vi "3.2.1-VectorNav WaitForReply.vi"(10 "error in":errorcluster, 11 "FPGA Ref In":T1) -> (2 "error out":errorcluster, 3 "FPGA Ref Out":T1)   [LabVIEW 2010]
doc: "In order for on-demand sampling to work, it's important that the cRIO and FPGA both agree on whether the FPGA should currently be sampling. This VI uses boolean flags to ensure that the FPGA knows when it's supposed to be sampling and that the cRIO knows when the FPGA is done so it can go grab the reply out of the Read FIFO."
uses:
  2-Low Neurons/2-FPGA VI Typedef.ctl
  2-Low Neurons/2.7-Sense Queries Typedef.ctl
  <vilib>/rvi/interface/nirviReadWriteControl/nirviReadWriteControl.xnode
  FPGA Bitfiles/DaveBrain_FPGATarget_1-Hindbrain_F0E489D8.lvbitx
  1-Hindbrain.vi
  <vilib>/rvi/interface/common/niFpgaNodeNameForErrorReporting.ctl
  <vilib>/rvi/errors/niLvFpgaWhatHappensToTopLevelVI.ctl
  2-Low Neurons/2.4-How Sensor Typedef.ctl
  <vilib>/Utility/error.llb/Error Cluster From Error Code.vi
  <vilib>/rvi/errors/niLvFpgaAdjustHostInterfaceError.vi
  3.0-Global.vi
  NiFpgaLv.dll
panel:
  out "VectorNav Ack Query":bool=TRUE
  out "VectorNav Cmd Query":bool=TRUE
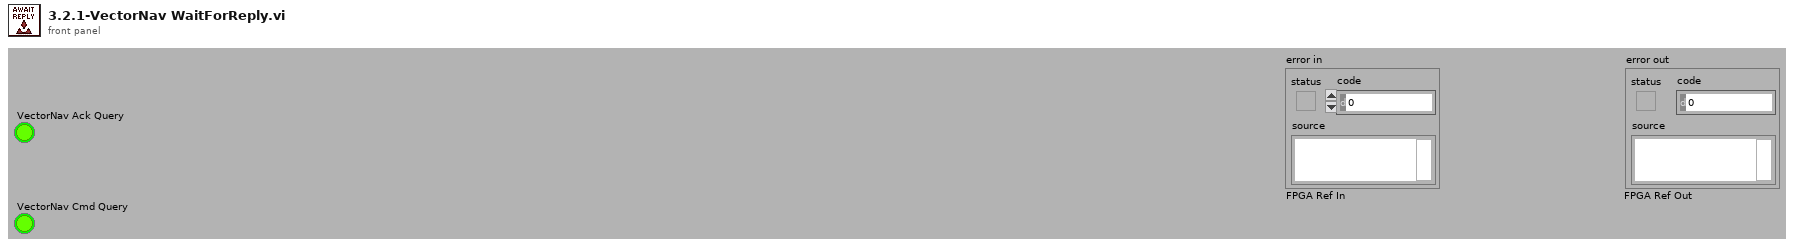
[diagram p1: front panel]
types:
  T1 = typedef "2-FPGA VI Typedef.ctl" = refnum<k20>
  T2 = typedef "2.7-Sense Queries Typedef.ctl" = cluster{"VectorNav Query":bool}
  T3 = typedef "niFpgaNodeNameForErrorReporting.ctl" = enum16{"Open FPGA VI Reference", "Read/Write Control", "Invoke Method: Abort", "Invoke Method: Acknowledge IRQ", "Invoke Method: Download", "Invoke Method: FIFO.Configure", "Invoke Method: FIFO.Read", "Invoke Method: FIFO.Start", "Invoke Method: FIFO.Stop", "Invoke Method: FIFO.Write", "Invoke Method: Reset", "Invoke Method: Run", "Invoke Method: Wait on IRQ", "Close FPGA VI Reference"}
  T4 = typedef "niLvFpgaWhatHappensToTopLevelVI.ctl" = enum16{"top level VI scripted behind XNode", "top level VI inlined behind XNode"}
  T5 = typedef "2.4-How Sensor Typedef.ctl" = cluster{"Motor Speed Integer":i32, "Drive Position Integer":i32, "Lidar Position Integer":i32, "Lidar Motor Position Integer":i32, "Steering Position Integer":i32, "Battery Voltage Fxp":fxp<+/-,16,5>, "Drive Encoder Cable Check":bool, "Lidar Drive Encoder Cable Check":bool, "Steer Encoder Cable Check":bool, "Lidar Pos Encoder Cable Check":bool, "Mod Buttons & Blinky Cable Check":bool, "Lidar Data Cable Check":bool, "Drive Motor Cable Check":bool, "Vector Nav Cable Check":bool, "Lidar Drive Cable Check":bool, "Steer Drive Cable Check":bool, "Reverse?":bool, "2.1  Steering Control Voltage":fxp<+/-,20,5>, "2.1 Drive Control Voltage":fxp<+/-,20,5>, "2.1  Lidar Control Voltage":fxp<+/-,20,5>, "2.5.7 A*B":fxp<+/-,18,1>, "2.1  Steering PID Output":fxp<+/-,20,5>, "2.1 Drive PID Output":fxp<+/-,20,5>, "2.1  Lidar PID Output":fxp<+/-,20,5>, "2.1.1 Drive Error":fxp<+/-,18,1>, "2.1.1 Drive Error I":fxp<+/-,64,46>, "2.1.1 Drive Error D":fxp<+/-,18,1>, "2.1.2 Steering Error":fxp<+/-,18,1>, "2.1.2 Steering Error I":fxp<+/-,64,46>, "2.1.2 Steering Error D":fxp<+/-,18,1>, "2.1.3 Lidar Error":fxp<+/-,18,1>, "2.1.3 Lidar Error I":fxp<+/-,64,46>, "2.1.3 Lidar Error D":fxp<+/-,18,1>, "VectorNav Ack Query":bool, "VectorNav Read Byte":u8, "VectorNav Read Status":enum16{"Waiting", "Reading", "Done"}}
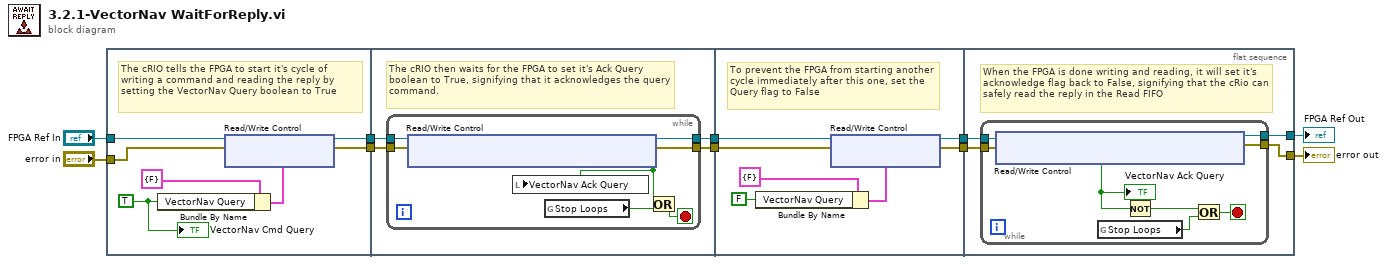
[diagram p0: block diagram]
diagram:
  n1 = flat-sequence {
    tunnel: [w17] -> w10
    tunnel: [w16] -> w9
    tunnel: "FPGA Ref In" -> [w12]
    tunnel: "error in" -> [w11]
    tunnel: w10 -> [w66]
    tunnel: [w65] -> w8
    tunnel: w9 -> [w64]
    tunnel: [w63] -> w7
    tunnel: w8 -> [w128]
    tunnel: [w125] -> w6
    tunnel: w7 -> [w127]
    tunnel: [w126] -> w5
    tunnel: w6 -> [w179]
    tunnel: w5 -> [w178]
    tunnel: [w177] -> w1
    tunnel: [w176] -> w3
    frame #0 {
      w14 = TRUE ("VectorNav-Query")
      # "The cRIO tells the FPGA to start it's cycle of writing a command and reading the reply by setting the VectorNav Query boolean to True"
      n2 = Bundle By Name(cluster=T2 {"VectorNav Query"=FALSE} ("2.7 Sense Queries"), "VectorNav Query"=w14) -> (w15:T2)
      n3 = xnode "Read/Write Control"("FPGA VI Reference In"=w12, "error in"=w11, "2.7 Sense Queries"=w15) -> ("FPGA VI Reference Out"=w17:T1, "error out"=w16:errorcluster)
      "VectorNav Cmd Query" <- w14
    }
    frame #1 {
      # "The cRIO then waits for the FPGA to set it's Ack Query boolean to True, signifying that it acknowledges the query command."
      n4 = while {
        tunnel: w66 -> [w72]
        tunnel: [w70] -> w65
        tunnel: w64 -> [w73]
        tunnel: [w71] -> w63
        stop <- w67 stop-if-true
        n5 = xnode "Read/Write Control"("FPGA VI Reference In"=w72, "error in"=w73) -> ("FPGA VI Reference Out"=w70:T1, "error out"=w71:errorcluster, "2.4 How Am I? Sensor.VectorNav Ack Query"=w68:bool)
        n6 = local write "VectorNav Ack Query"(w68) -> ()
        n7 = global read "3.0-Global.vi" "Stop Loops"() -> (w69:bool)
        n8 = Or(x=w68, y=w69) -> (x .or. y?=w67:bool)
      }
    }
    frame #2 {
      # "To prevent the FPGA from starting another cycle immediately after this one, set the Query flag to False"
      n9 = Bundle By Name(cluster=T2 {"VectorNav Query"=FALSE} ("2.7 Sense Queries"), "VectorNav Query"=FALSE) -> (w130:T2)
      n10 = xnode "Read/Write Control"("FPGA VI Reference In"=w128, "error in"=w127, "2.7 Sense Queries"=w130) -> ("FPGA VI Reference Out"=w125:T1, "error out"=w126:errorcluster)
    }
    frame #3 {
      # "When the FPGA is done writing and reading, it will set it's acknowledge flag back to False, signifying that the cRio can safely read the reply in the Read FIFO"
      n11 = while {
        tunnel: w179 -> [w187]
        tunnel: w178 -> [w186]
        tunnel: [w185] -> w177
        tunnel: [w184] -> w176
        stop <- w180 stop-if-true
        n12 = xnode "Read/Write Control"("FPGA VI Reference In"=w187, "error in"=w186) -> ("FPGA VI Reference Out"=w185:T1, "error out"=w184:errorcluster, "2.4 How Am I? Sensor.VectorNav Ack Query"=w183:bool)
        "VectorNav Ack Query" <- w183
        n13 = global read "3.0-Global.vi" "Stop Loops"() -> (w181:bool)
        n14 = Not(x=w183) -> (.not. x?=w182:bool)
        n15 = Or(x=w182, y=w181) -> (x .or. y?=w180:bool)
      }
    }
  }
  "error out" <- w3
  "FPGA Ref Out" <- w1
